vi "Day 23 - Unstable Diffusion.vi"() -> ()   [LabVIEW 2020, in "AoC 2022.lvlib"]
uses:
  AoC 2022.lvlib
  345cb393-b29b-40d9-8f2b-ec06807a071d.vi
  35999f4b-5669-428c-b693-a448302dda71.vi
  5a7c10e5-125f-4244-8cca-a7389e644c3c.vi
  a5048498-a69e-44af-a810-29afce3209e7.vi
  bd3f67bb-b31b-4699-b773-9a91305869c5.vi
  6851dff7-3c12-4484-a5dc-fd25fc653725.vi
  351d0007-024e-4366-aac0-d32e01098aac.vi
  9af85e8f-27f2-4200-b2e6-dc1860d62b81.vi
panel:
  out "Elves Sonar":cluster{T1[]}[](graph)
  out "#Rounds Ended":i32
  in  "millisecond multiple":u32=20
  in  "Puzzle Input":string="....#..\n..###.#\n#...#.#\n.#...##\n#.###..\n##.#.##\n.#..#.."
  out "Puzzle Answer":string
  # "Puzzle Part-2 Answer"
  # "Press Ctrl+M & Enter the Puzzle Input and run the VI"
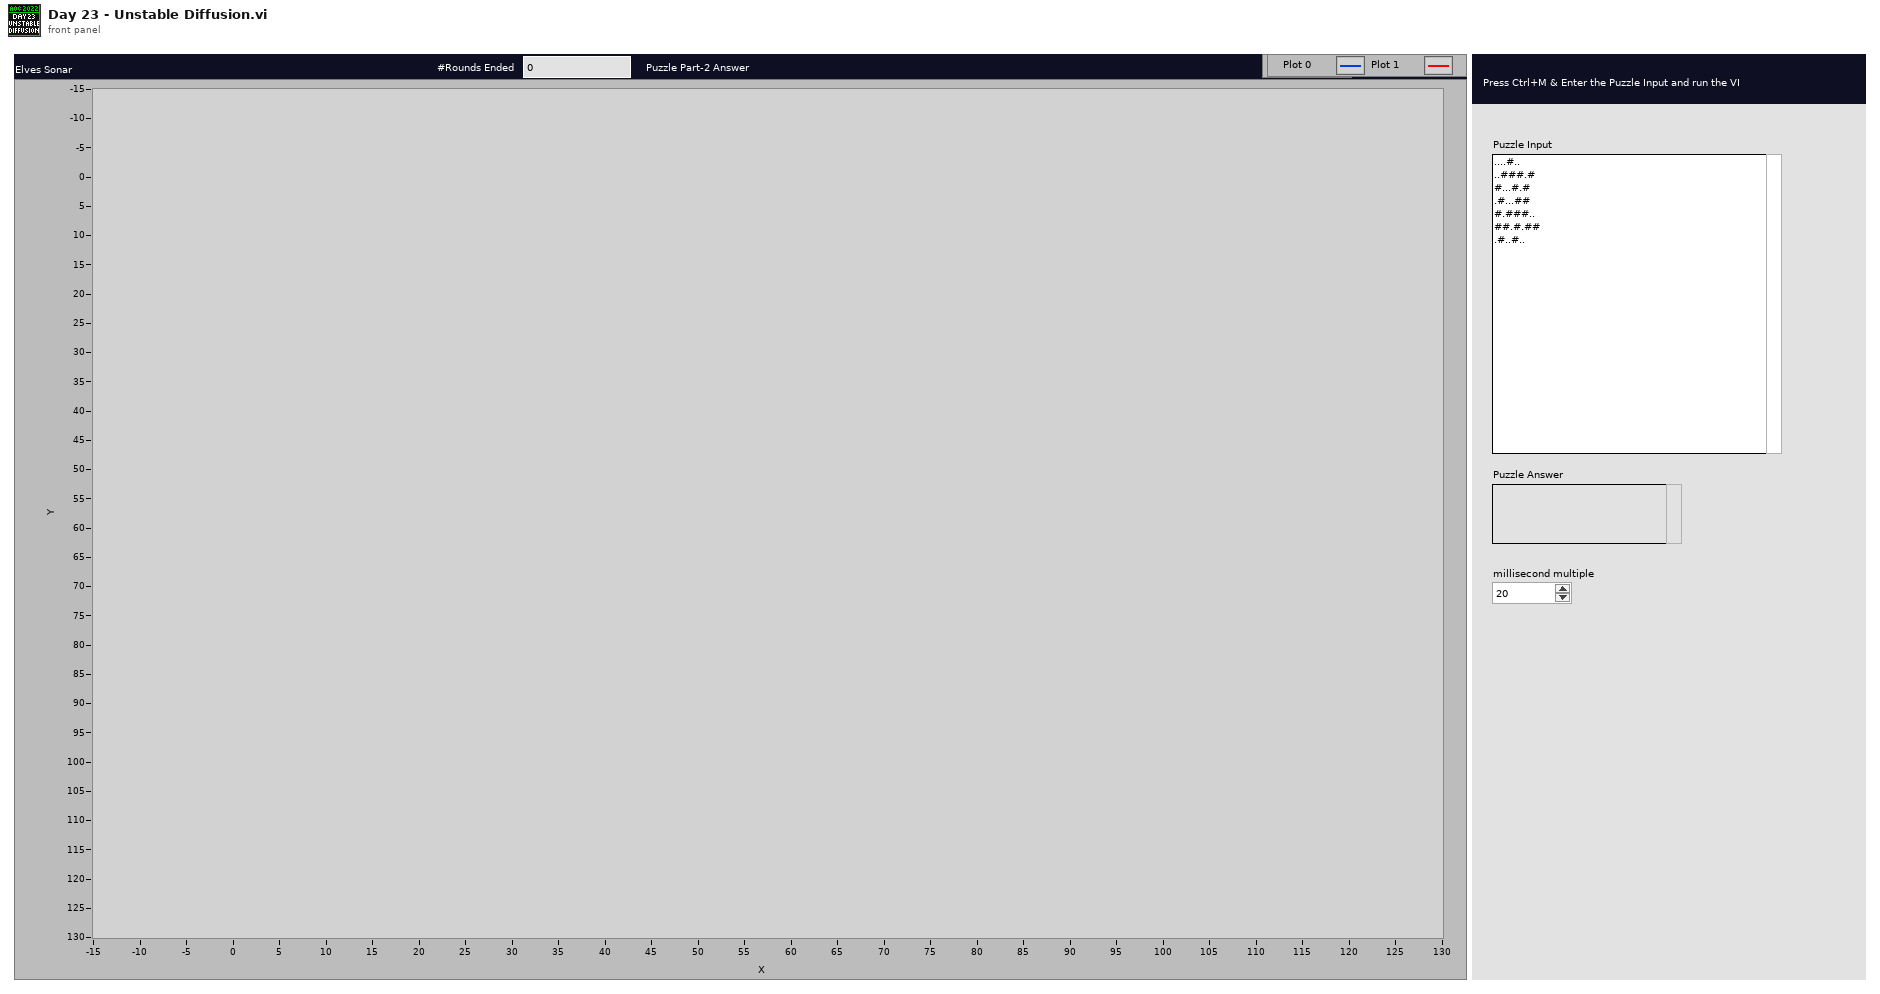
[diagram p1: front panel]
types:
  T1 = typedef "AoC 2022.lvlib/Location.ctl" = cluster{"X":i32, "Y":i32}
  T2 = cluster{"Has any Empty Space ?":T1[], "Move":T1}[]
  T3 = map{T1, cluster{"Has any Empty Space ?":T1[], "Move":T1}[]}
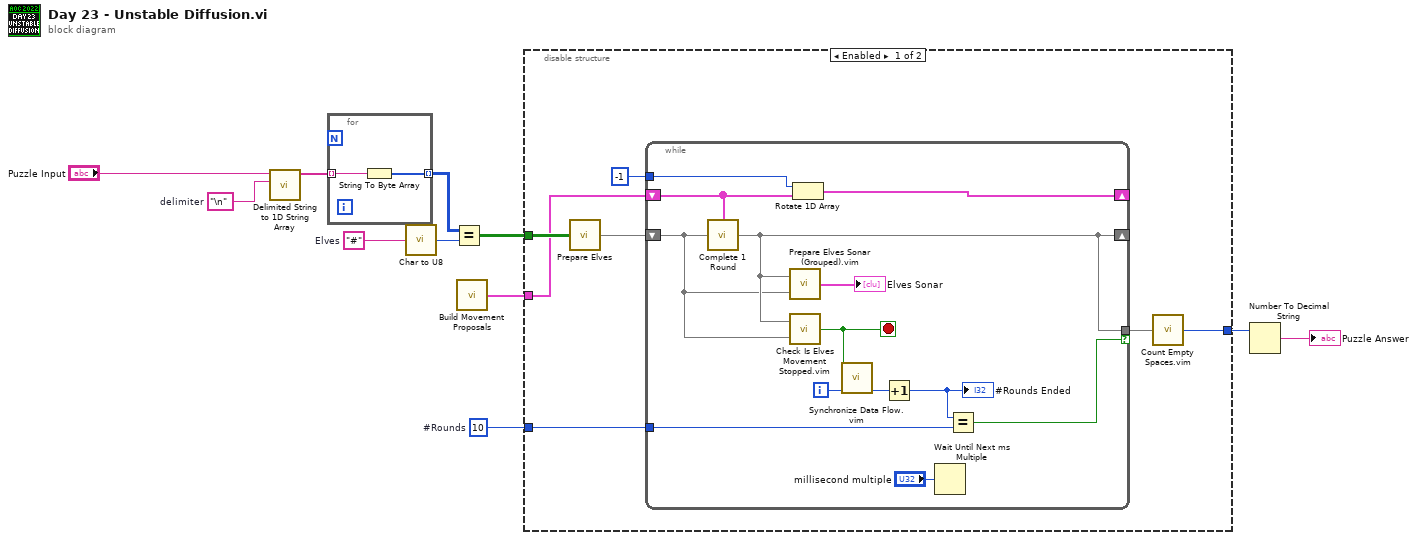
[diagram p0: block diagram]
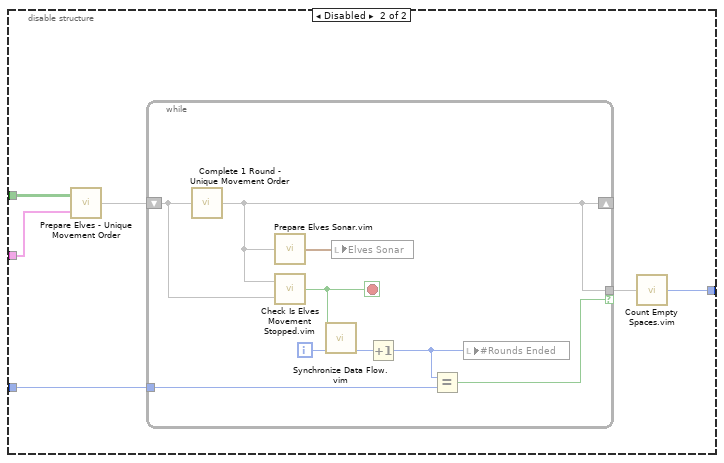
[diagram p2: hidden frame]
diagram:
  w1 = 10  # #Rounds
  w7 = "#"  # Elves
  w9 = "\n"  # delimiter
  n1 = call <vilib>:"Delimited String to 1D String Array.vi"("delimiter"=w9, "delimited string"="Puzzle Input") -> ("string array"=w8:string[])  [unwired: 9 in]
  n2 = for {
    tunnel: w8 -> [w13] mode=indexing
    tunnel: [w12] -> w5 mode=indexing
    n3 = String To Byte Array(string=w13) -> (unsigned byte array=w12:u8[])
  }
  n4 = call "Char to U8.vi"("Char"=w7) -> ("U8"=w6:u8)
  n5 = Equal?(x=w5, y=w6) -> (x = y?=w2:bool[][])
  n6 = call "Build Movement Proposals.vi"() -> ("Movement Proposal Rules"=w4:T2)
  n7 = disable-structure shown="Enabled" {
    disable-tunnel: w4 -> [w15 w39]
    disable-tunnel: [w20 w37] -> w3
    disable-tunnel: w2 -> [w17 w36]
    disable-tunnel: w1 -> [w18 w34]
    frame Enabled {
      n8 = call "Prepare Elves.vi"("Elves' Sonar"=w17) -> ("Elves"=w16:set{T1})
      n9 = while {
        shift-right: [w32] -> _
        shift-left: w16 -> [w22]
        tunnel: [w32] -> w19 if=w26
        tunnel: w18 -> [w28]
        shift-right: [w24] -> _
        shift-left: w15 -> [w25]
        tunnel: -1 -> [w23]
        i -> [w30]
        stop <- w31 stop-if-true
        n10 = call "Complete 1 Round.vi"("Elves in"=w22, "Movement Proposal Rules"=w25) -> ("Elves out"=w32:set{T1})
        n11 = call "Prepare Elves Sonar (Grouped).vim"("Elves Previous State"=w22, "Elves Current State"=w32) -> ("Elves Sonar"=→"Elves Sonar":cluster{T1[]}[])
        n12 = call "Check Is Elves Movement Stopped.vim"("Elves' Previous State"=w22, "Elves' Current State"=w32) -> ("No Movement ?"=w31:bool)
        n13 = Rotate 1D Array(1:w25, 2:w23) -> (0:w24:T2)
        n14 = call "Synchronize Data Flow.vim"("input 4"=w30, "input 1"=w31) -> ("output 4"=w29:i32)  [unwired: 2 in, 3 out]
        n15 = Increment(x=w29) -> (x+1=w27:i32)
        "#Rounds Ended" <- w27
        n16 = Wait Until Next ms Multiple(millisecond multiple="millisecond multiple") -> ()  [unwired: 1 out]
        n17 = Equal?(x=w27, y=w28) -> (x = y?=w26:bool)
      }
      n18 = call "Count Empty Spaces.vim"("Elves with Unique Movement Order"=w19) -> ("#Empty Spaces"=w20:i16)
    }
    frame Disabled {
      n19 = call "Prepare Elves - Unique Movement Order.vi"("Movement Proposal Rules"=w39, "Elves' Positions"=w36) -> ("Elves with Unique Movement Order"=w38:T3)
      n20 = while {
        shift-right: [w47] -> _
        shift-left: w38 -> [w48]
        tunnel: [w47] -> w35 if=w42
        tunnel: w34 -> [w43]
        i -> [w45]
        stop <- w46 stop-if-true
        n21 = call "Complete 1 Round - Unique Movement Order.vi"("Elves in"=w48) -> ("Elves out"=w47:T3)
        n22 = call "Prepare Elves Sonar.vim"("Elves"=w47) -> ("Elves Sonar"=w41:T1[])
        n23 = call "Check Is Elves Movement Stopped.vim"("Elves' Previous State"=w48, "Elves' Current State"=w47) -> ("No Movement ?"=w46:bool)
        n24 = call "Synchronize Data Flow.vim"("input 4"=w45, "input 1"=w46) -> ("output 4"=w44:i32)  [unwired: 2 in, 3 out]
        n25 = local write "Elves Sonar"(w41) -> ()
        n26 = Increment(x=w44) -> (x+1=w40:i32)
        n27 = Equal?(x=w40, y=w43) -> (x = y?=w42:bool)
        n28 = local write "#Rounds Ended"(w40) -> ()
      }
      n29 = call "Count Empty Spaces.vim"("Elves with Unique Movement Order"=w35) -> ("#Empty Spaces"=w37:i16)
    }
  }
  n30 = Number To Decimal String(number=w3) -> (decimal integer string=→"Puzzle Answer":string)  [unwired: 1 in]
